vi "Fault -Injection Test.vi"() -> ()   [LabVIEW 2021]
uses:
  Source/Fault-Injection Bus/Support/Value Type/Boolean/Support/Value Type.ctl
  Source/Fault-Injection Bus/Support/Value Type/SGL/Support/Value Type.ctl
  Source/Omni-Bus/Omni_Bus.lvclass
  Source/Omni-Bus/Support/Broad Types.ctl
  Source/Local Bus/Local Bus.lvclass
  C:/Users/Tim/Documents/GitHub/Omni-Bus/Source/Omni-Bus/Bus Access/Bus_Access.lvclass
  <vilib>/Utility/Data Type/Type Definitions/Data Type.ctl
  Source/Fault-Injection Bus/Fault-Injection Bus.lvclass
  <vilib>/TSA/Abstract Data Classes/Abs_Types/Type/Abs_Type.lvclass/Abs_Type.ctl
  Source/Omni-Bus/Omni_Bus.lvclass/Omni_Bus.ctl
  Source/Omni-Bus/Support/Write/Write DBL.vi
  Source/Omni-Bus/Support/Get/Static/Get Static SGL.vi
  Source/Omni-Bus/Support/Get/Static/Get Static Boolean.vi
  Source/Omni-Bus/Support/Read/Read SGL.vi
  Source/Omni-Bus/Support/Read/Read Multi Boolean.vi
  Source/Omni-Bus/Support/Read/Read DBL.vi
  Source/Omni-Bus/Support/Get/Get DBL.vi
  Source/Omni-Bus/Support/FindVar.vi
  Source/Omni-Bus/Support/Get/Get Multi Boolean.vi
  Source/Omni-Bus/Support/Get/Get SGL.vi
  <vilib>/Utility/error.llb/Clear Errors.vi
  Source/Omni-Bus/Properties/Read Var Map.vi
  <vilib>/TSA/Abstract Data Classes/Abs_Types/Type/Properties/Read Tag.vi
  Source/Omni-Bus/Support/FindMultiVar.vi
  <vilib>/TSA/Abstract Data Classes/Abs_Types/Double Float/Abs_Double Float.lvclass
  C:/Program Files (x86)/National Instruments/LabVIEW 2021/vi.lib/TSA/Abstract Data Classes/Abs_Types/Type/Abs_Type.lvclass
  <vilib>/TSA/Abstract Data Classes/Abs_Types/Value/Abs_Value.lvclass
  Source/Fault-Injection Bus/Support/Value Type/DBL/Fault-Injection_DBL.lvclass
  Source/Fault-Injection Bus/Support/Value Type/SGL/Fault-Injection_SGL.lvclass
  C:/Program Files (x86)/National Instruments/LabVIEW 2021/vi.lib/TSA/Abstract Data Classes/Abs_Types/Single Float/Abs_Single Float.lvclass
  C:/Program Files (x86)/National Instruments/LabVIEW 2021/vi.lib/TSA/Abstract Data Classes/Abs_Types/Value/Abs_Value.lvclass
  <vilib>/TSA/Abstract Data Classes/Abs_Types/Single Float/Abs_Single Float.lvclass
  Source/Fault-Injection Bus/Support/Value Type/Boolean/Fault-Injection_Boolean.lvclass
  C:/Program Files (x86)/National Instruments/LabVIEW 2021/vi.lib/TSA/Abstract Data Classes/Abs_Types/Boolean/Abs_Boolean.lvclass
  <vilib>/TSA/Abstract Data Classes/Abs_Types/Boolean/Abs_Boolean.lvclass
  Source/Omni-Bus/Support/Check For Read Only Error.vi
  Source/Omni-Bus/Support/Incorrect Tag String Error.vi
  <vilib>/TSA/Abstract Data Classes/Abs_Types/Single Float/Static Write.vi
  <vilib>/TSA/Abstract Data Classes/Abs_Types/Type/Abs_Type.lvclass
  <vilib>/Utility/Data Type/NI_Data Type.lvlib
  Source/Fault-Injection Bus/Support/Interfaces/Type/Fault-Injection_Type.lvclass
  C:/Users/Tim/Documents/GitHub/Omni-Bus/Source/Fault-Injection Bus/Support/Value Type/Boolean/Fault-Injection_Boolean.lvclass
  C:/Users/Tim/Documents/GitHub/Omni-Bus/Source/Fault-Injection Bus/Support/Interfaces/Type/Fault-Injection_Type.lvclass
  C:/Program Files (x86)/National Instruments/LabVIEW 2021/vi.lib/TSA/Abstract Data Classes/Abs_Types/Floating Point/Abs_Floating Point.lvclass
  C:/Program Files (x86)/National Instruments/LabVIEW 2021/vi.lib/TSA/Abstract Data Classes/Abs_Types/Numeric/Abs_Numeric.lvclass
  C:/Users/Tim/Documents/GitHub/Omni-Bus/Source/Fault-Injection Bus/Support/Interfaces/SGL/Fault-Injection_SGL_Type.lvclass
  C:/Users/Tim/Documents/GitHub/Omni-Bus/Source/Fault-Injection Bus/Support/Value Type/SGL/Fault-Injection_SGL.lvclass
panel:
  out "error out 6":errorcluster
  in  "Enable 3":bool
  in  "Injected Value 2":dbl
  out "Numeric 2":dbl
  in  "Value 3":dbl
  in  "Injected Value":T1
  in  "Value":sgl
  out "error out 5":errorcluster
  in  "Enable":bool
  out "Numeric":sgl
  in  "Enable 2":T2
  in  "Value 2":T2
  in  "Tag 4":string(combo)
  out "error out 4":errorcluster
  in  "Arm":bool
  in  "Array":bool[](array[boolean])
  out "Booleans":bool[](array[boolean])
  out "error out 3":errorcluster
  out "error out 2":errorcluster
  in  "Tag 2":string[](array[combo])
  in  "stop":bool
  in  "Tags":string[](array[combo])
  out "error out":errorcluster
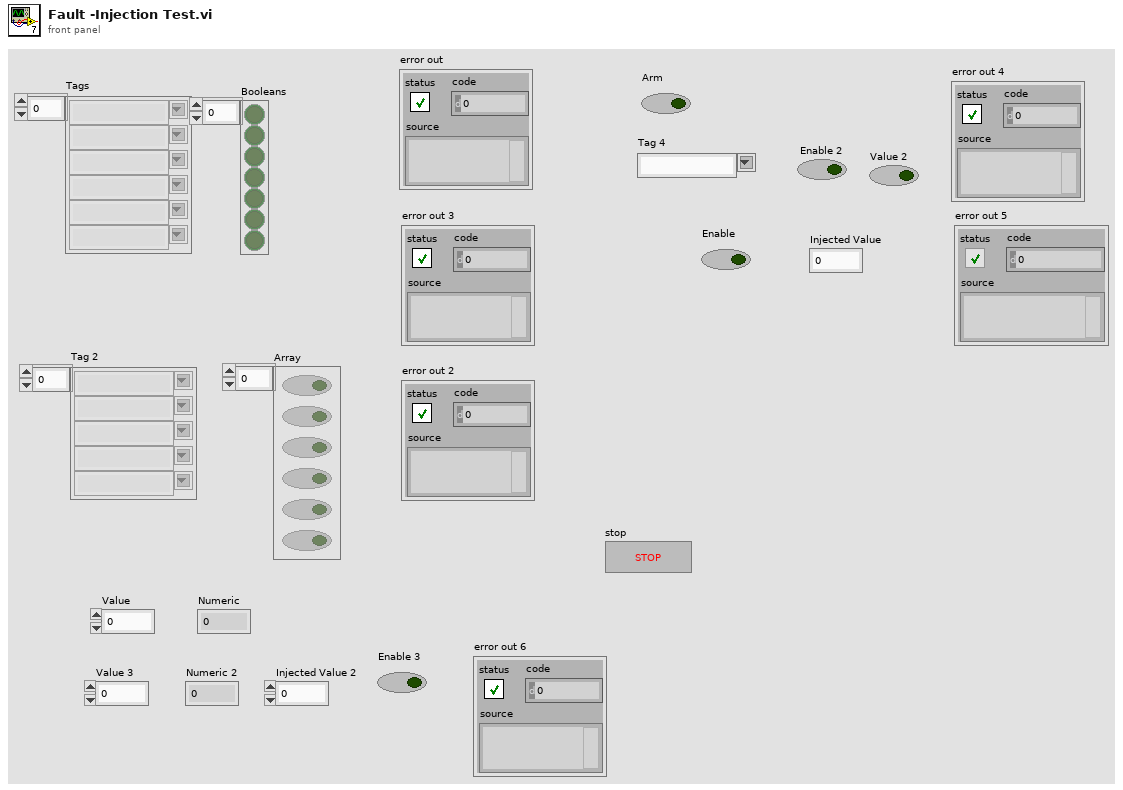
[diagram p1: front panel]
types:
  T1 = typedef "Fault-Injection_SGL.lvclass/Value Type.ctl" = sgl
  T2 = typedef "Fault-Injection_Boolean.lvclass/Value Type.ctl" = bool
  T3 = typedef "NI_Data Type.lvlib/Data Type.ctl" = enum8{"Invalid Type", "Void", "I8", "I16", "I32", "I64", "U8", "U16", "U32", "U64", "Single Float", "Double Float", "Extended Float", "Single Complex", "Double Complex", "Extended Complex", "Enum U8", "Enum U16", "Enum U32", "Enum U64", "Single Float With Unit", "Double Float With Unit", "Extended Float With Unit", "Single Complex with Unit", "Double Complex with Unit", "Extended Complex with Unit", "Boolean", "String", "Path", "Picture", "Tag", "Array", "Cluster", "Variant", "LV Variant", "Waveform", "Timestamp", "Digital Waveform", "Digital Data", "ExpressData", "Refnum", "External Data", "VI", "Poly VI", "LabVIEW Class Instance", "Fixed Point", "Set Collection", "Map Collection"}
  T4 = typedef "Omni_Bus.lvclass/Broad Types.ctl" = enum16{"All Tags", "NI Specific Type", "Boolean", "String", "Numeric", "Float", "Integer", "Collection", "All Value Types", "Non Value Types"}
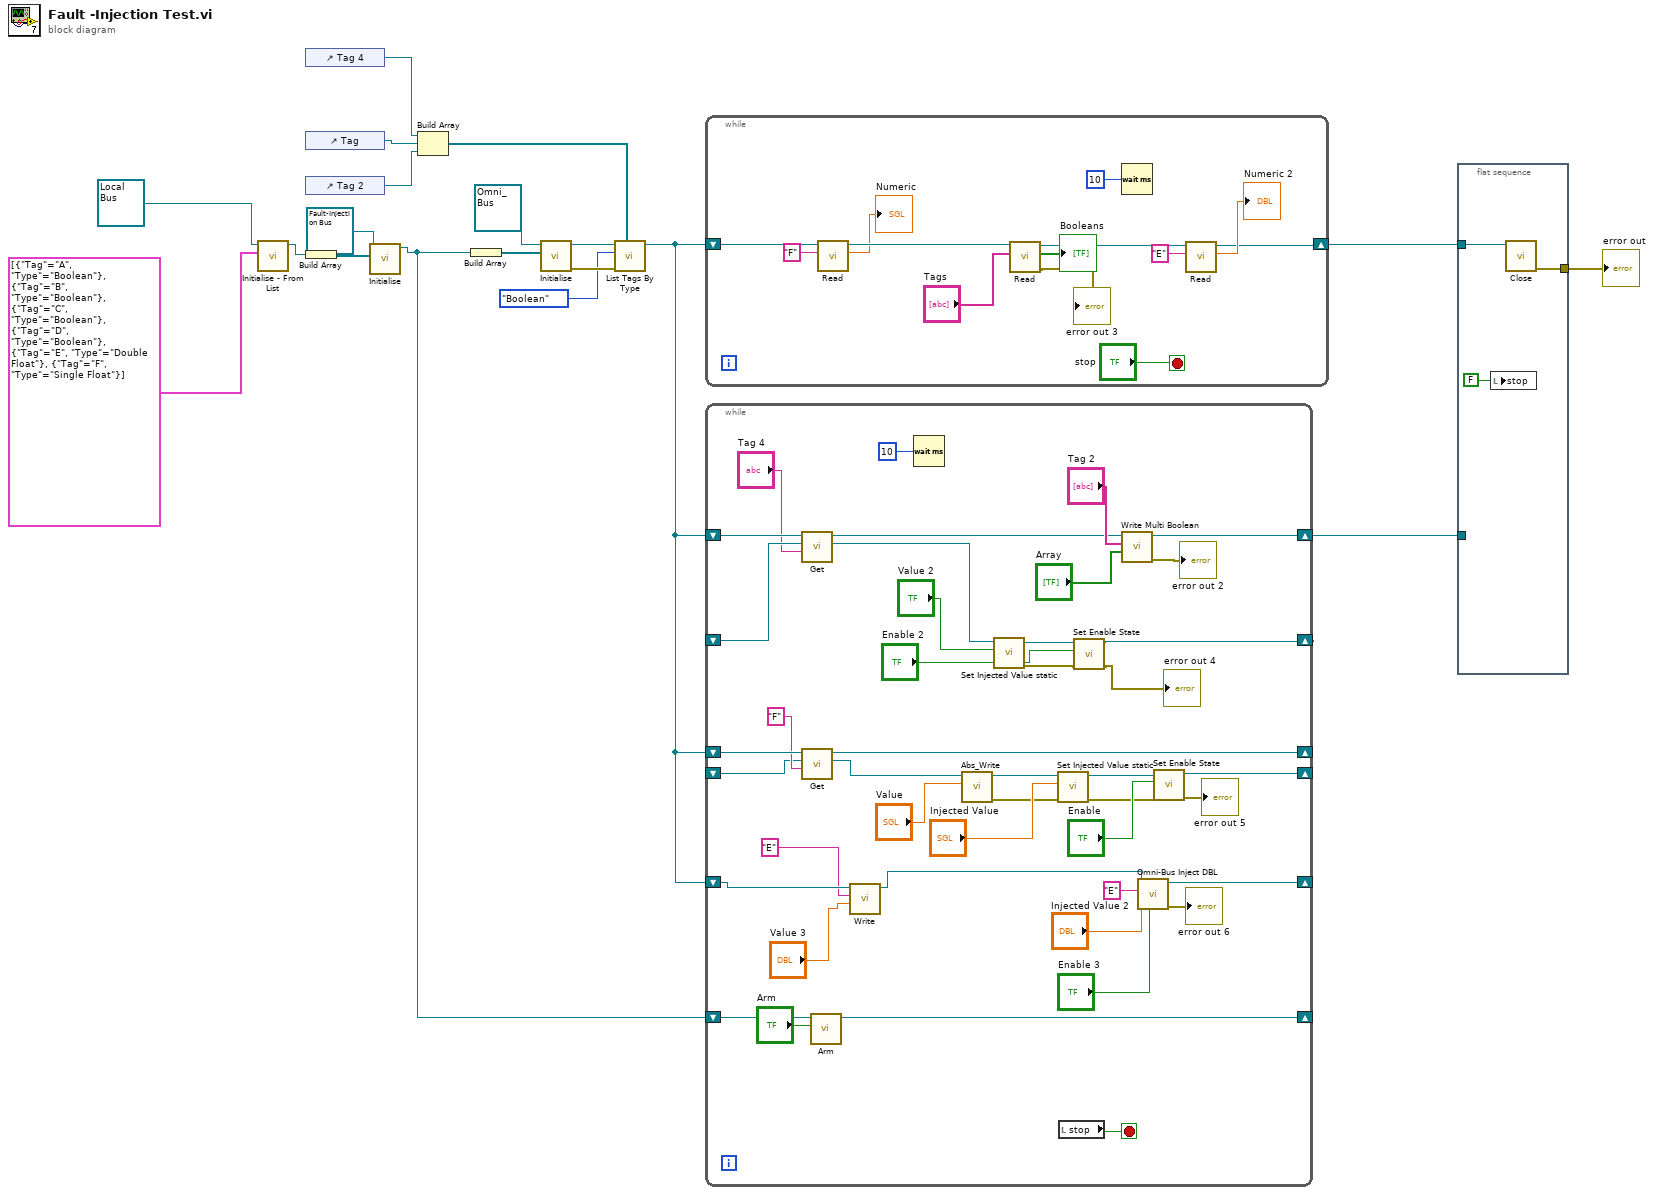
[diagram p0: block diagram]
diagram:
  n1 = call "Initialise - From List.vi"("Tag List"=cluster{"Tag":string, "Type":T3}[] [{"Tag"="A", "Type"=enum."Boolean"}, {"Tag"="B", "Type"=enum."Boolean"}, {"Tag"="C", "Type"=enum."Boolean"}, {"Tag"="D", "Type"=enum."Boolean"}, {"Tag"="E", "Type"=enum."Double Float"}, {"Tag"="F", "Type"=enum."Single Float"}], "Local Bus in"=refnum<class "Local Bus.lvclass"> refnum ("Local Bus.lvclass")) -> ("Local Bus out"=w6:refnum<class "Local Bus.lvclass">)  [unwired: 8 in, 1 out]
  n2 = control-ref of="Tag 4"() -> (w2:refnum<vi>)
  n3 = control-ref of="Tag"() -> (w9:refnum<vi>)
  n4 = control-ref of="Tag 2"() -> (w8:refnum<vi>)
  n5 = Build Array(w6) -> (w5:refnum<class "Local Bus.lvclass">[])
  n6 = call "Initialise.vi"("Buses"=w5, "Fault-Injection Bus in"=refnum<class "Fault-Injection Bus.lvclass"> refnum) -> ("Fault-Injection Bus out"=w3:refnum<class "Fault-Injection Bus.lvclass">)  [unwired: 8 in, 1 out]
  n7 = Build Array(w2, w9, w8) -> (w7:refnum<vi>[])
  n8 = Build Array(w3) -> (w18:refnum<class "Fault-Injection Bus.lvclass">[])
  n9 = call-dynamic "Initialise.vi"("Bus Access"=w18, "Var Bus in"=refnum<class "Omni_Bus.lvclass"> refnum) -> ("error out"=w16:errorcluster, "Var Bus out"=w17:refnum<class "Omni_Bus.lvclass">)  [unwired: 8 in]
  n10 = call "List Tags By Type.vi"("Combo Boxes"=w7, "error in (no error)"=w16, "Broad Types"=Broad_Types."Boolean", "Var Bus in"=w17) -> ("Var Bus out"=w1:refnum<class "Omni_Bus.lvclass">)  [unwired: 4 in, 3 out]
  n11 = while {
    shift-right: [w20] -> w13
    shift-left: w1 -> [w27]
    stop <- "stop" stop-if-true
    n12 = call-poly "Read.vi"("Tag"="F", "Var Bus in"=w27) -> ("Numeric"=→"Numeric":sgl, "Var Bus out"=w26:refnum<class "Omni_Bus.lvclass">)  [unwired: 7 in, 1 out]
    n13 = call-poly "Read.vi"("Tags"="Tags", "Var Bus in"=w26) -> ("error out"=→"error out 3":errorcluster, "Booleans"=→"Booleans":bool[], "Var Bus out"=w21:refnum<class "Omni_Bus.lvclass">)  [unwired: 7 in]
    n14 = Wait (ms)(milliseconds to wait=u32 10) -> ()  [unwired: 1 out]
    n15 = call-poly "Read.vi"("Tag"="E", "Var Bus in"=w21) -> ("Numeric"=→"Numeric 2":dbl, "Var Bus out"=w20:refnum<class "Omni_Bus.lvclass">)  [unwired: 7 in, 1 out]
  }
  n16 = while {
    shift-right: [w73] -> w12
    shift-left: w1 -> [w66]
    shift-right: [w67] -> _
    shift-left: w3 -> [w69]
    shift-right: [w60] -> _
    shift-left: _ -> [w64]
    shift-right: [w54] -> _
    shift-left: w1 -> [w55]
    shift-right: [w51] -> _
    shift-left: _ -> [w52]
    shift-right: [w40] -> _
    shift-left: w1 -> [w37]
    stop <- w75 stop-if-true
    n17 = call-poly "Get.vi"("Tag"="Tag 4", "Value Type"=w64, "Var Bus in"=w66) -> ("Value Out"=w62:refnum<class "Fault-Injection_Boolean.lvclass">, "Var Bus out"=w65:refnum<class "Omni_Bus.lvclass">)  [unwired: 5 in, 2 out]
    n18 = call-poly "Get.vi"("Tag"="F", "Value Type"=w52, "Var Bus in"=w55) -> ("Value Out"=w48:refnum<class "Fault-Injection_SGL.lvclass">, "Var Bus out"=w54:refnum<class "Omni_Bus.lvclass">)  [unwired: 5 in, 2 out]
    n19 = call "Arm.vi"("Arm"="Arm", "Fault-Injection Bus in"=w69) -> ("Fault-Injection Bus out"=w67:refnum<class "Fault-Injection Bus.lvclass">)  [unwired: 8 in, 1 out]
    n20 = call-poly "Write.vi"("Numeric"="Value 3", "Tag"="E", "Omni_Bus in"=w37) -> ("Omni_Bus out"=w36:refnum<class "Omni_Bus.lvclass">)  [unwired: 7 in, 1 out]
    n21 = Wait (ms)(milliseconds to wait=u32 10) -> ()  [unwired: 1 out]
    n22 = call-poly <vilib>:"Abs_Write.vi"("Value"="Value", "Abs_Single Float in"=w48) -> ("error out"=w42:errorcluster, "Abs_Single Float out"=w46:refnum<class "Fault-Injection_SGL.lvclass">)  [unwired: 8 in]
    n23 = call "Set Injected Value static.vi"("Value"="Value 2", "Fault-Injection_Boolean in"=w62) -> ("error out"=w59:errorcluster, "Fault-Injection_Boolean out"=w56:refnum<class "Fault-Injection_Boolean.lvclass">)  [unwired: 8 in]
    n24 = call "Set Injected Value static.vi"("error in (no error)"=w42, "Value"="Injected Value", "Fault-Injection_Boolean in"=w46) -> ("error out"=w43:errorcluster, "Fault-Injection_Boolean out"=w45:refnum<class "Fault-Injection_SGL.lvclass">)  [unwired: 7 in]
    n25 = local read "stop"() -> (w75:bool)
    n26 = call "Set Enable State.vi"("error in (no error)"=w59, "Enable"="Enable 2", "Abs_Value.lvclass in"=w56) -> ("error out"=→"error out 4":errorcluster, "Abs_Value.lvclass out"=w60:refnum<class "Fault-Injection_Boolean.lvclass">)  [unwired: 7 in]
    n27 = call "Write Multi Boolean.vi"("Array"="Array", "Tag"="Tag 2", "Omni_Bus in"=w65) -> ("error out"=→"error out 2":errorcluster, "Omni_Bus out"=w73:refnum<class "Omni_Bus.lvclass">)  [unwired: 7 in]
    n28 = call "Omni-Bus Inject DBL.vi"("Enable"="Enable 3", "Injected Value"="Injected Value 2", "Tag"="E", "Omni_Bus in"=w36) -> ("error out"=→"error out 6":errorcluster, "Omni_Bus out"=w40:refnum<class "Omni_Bus.lvclass">)  [unwired: 6 in]
    n29 = call "Set Enable State.vi"("error in (no error)"=w43, "Enable"="Enable", "Abs_Value.lvclass in"=w45) -> ("error out"=→"error out 5":errorcluster, "Abs_Value.lvclass out"=w51:refnum<class "Fault-Injection_SGL.lvclass">)  [unwired: 7 in]
  }
  n30 = flat-sequence {
    tunnel: [w78] -> w14
    tunnel: w13 -> [w77]
    tunnel: w12 -> [_]
    frame #0 {
      n31 = local write "stop"(FALSE ("stop")) -> ()
      n32 = call-dynamic "Close.vi"("Data in"=w77) -> ("error out"=w78:errorcluster)  [unwired: 9 in, 1 out]
    }
  }
  "error out" <- w14
